vi "Test.lua.vi"(0 "L":u64, 1 "Lua Dll":path) -> ()   [LabVIEW 2014]
uses:
  <vilib>/Utility/VariantDataType/Type.ctl
  <vilib>/Utility/VariantDataType/VariantType.lvlib
panel:
  out "data":variant[][](array[variant])
  out "Variant":variant
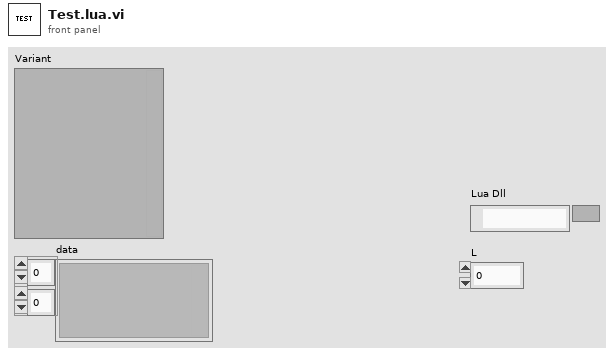
[diagram p1: front panel]
types:
  T1 = typedef "VariantType.lvlib/Type.ctl" = enum8{"Invalid Type", "Void", "I8", "I16", "I32", "I64", "U8", "U16", "U32", "U64", "Single Float", "Double Float", "Extended Float", "Single Complex", "Double Complex", "Extended Complex", "Enum U8", "Enum U16", "Enum U32", "Enum U64", "Single Float With Unit", "Double Float With Unit", "Extended Float With Unit", "Single Complex with Unit", "Double Complex with Unit", "Extended Complex with Unit", "Boolean", "String", "Path", "Picture", "Tag", "Array", "Cluster", "Variant", "LV Variant", "Waveform", "Timestamp", "Digital Waveform", "Digital Data", "ExpressData", "Refnum", "External Data", "VI", "Poly VI", "LabVIEW Class Instance", "Fixed Point"}
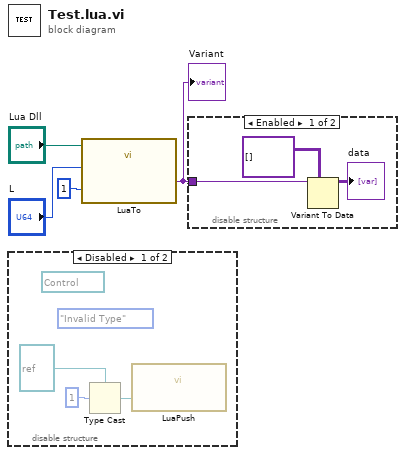
[diagram p0: block diagram]
diagram:
  n1 = disable-structure shown="Disabled" {
    frame Disabled {
      (unwired) Type."Invalid Type" ("Type Enum")
      (unwired) refnum<vi> refnum ("reference")
      n2 = Type Cast(type=refnum<vi> refnum ("vi reference"), x=1) -> (*(type *) &x=w6:refnum<vi>)
      n3 = call "LuaPush.vi"("Variant"=w6) -> ()  [unwired: 2 in, 1 out]
    }
    frame Enabled {
    }
  }
  n4 = call "LuaTo.vi"("Index"=1 ("n"), "L In"="L", "Lua Dll"="Lua Dll") -> ("Variant"=w2:variant)  [unwired: 5 out]
  "Variant" <- w2
  n5 = disable-structure shown="Enabled" {
    disable-tunnel: w2 -> [w9 _]
    frame Enabled {
      n6 = Variant To Data(type=variant[][] [], Variant=w9) -> (data=→"data":variant[][])  [unwired: 1 in, 1 out]
    }
    frame Disabled {
    }
  }
